vi "Pre Launch Init.vi"(11 "IMAQdx Cam Actor in":refnum<class "IMAQdx Cam Actor.lvclass">) -> (0 "error out":errorcluster, 3 "IMAQdx Cam Actor out":refnum<class "IMAQdx Cam Actor.lvclass">)   [LabVIEW 2014, in "IMAQdx Cam Actor.lvlib" / "IMAQdx Cam Actor.lvclass"]
doc: "(<B>Filename</B>: Actor Framework.lvlib:Actor.lvclass:Pre Launch Init.vi)\n\nDefines behavior that occurs after the Launch Nested Actor method is invoked but before the actor's Actor Core method begins running.\n\nBy default, this method does nothing. A descendant class may override it to define behavior."
uses:
  IMAQdx Cam Actor.lvclass
  <vilib>/ActorFramework/Actor/Actor.lvclass
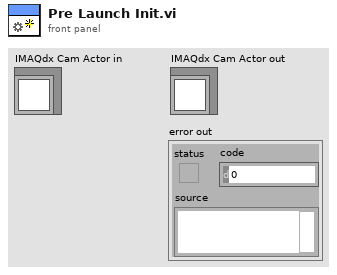
[diagram p1: front panel]
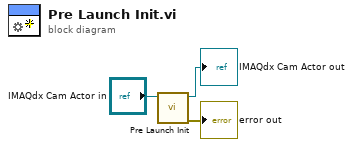
[diagram p0: block diagram]
diagram:
  n1 = call-parent "Pre Launch Init.vi"("Actor in"="IMAQdx Cam Actor in") -> ("error out"=→"error out":errorcluster, "Actor out"=→"IMAQdx Cam Actor out":refnum<class "IMAQdx Cam Actor.lvclass">)  [unwired: 9 in]
